vi "line-follower.vi"() -> ()   [LabVIEW 2016]
uses:
  <vilib>/NXT/Block Support/NXT_InputPort.ctl
  <vilib>/NXT/Block Support/NXT_OutputPort.ctl
  <vilib>/NXT/NXTIO Xnodes/NXTIONodeSubVIs/NXTMoveMotors.vi
  <vilib>/NXT/Dual Mode Library/Sensors/EV3_Color_Reflect.vi
  <vilib>/NXT/Dual Mode Library/Waits/Wait_Num(msec).vi
  <vilib>/NXT/NXTIO Xnodes/NXTIONodeSubVIs/NXTStopMotors.vi
  <vilib>/NXT/Dual Mode Library/Waits/Wait_LetGo.vi
  <vilib>/NXT/Dual Mode Library/Waits/Wait_Bump.vi
  <vilib>/NXT/Dual Mode Library/Display/drawText.vi
  <vilib>/NXT/Dual Mode Library/Sensors/Touch_Pressed.vi
  <vilib>/NXT/NXTIO Xnodes/AddressXNode/NXTIOAddress.xnode
  <vilib>/NXT/Subs/LVHSConnector.ctl
  <vilib>/NXT/NXTIO Xnodes/NXTIOXNode/NXTIO.xnode
  <vilib>/NXT/LegoClasses/BrickReference/BrickReference.lvclass
panel:
  out "Counter":sgl
  out "Y":dbl
  out "E":sgl
  out "X":sgl
  out "Motor B":dbl
  out "Motor A":dbl
  out "Avg":sgl
  out "max":sgl
  out "min":sgl
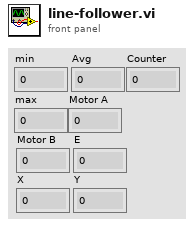
[diagram p1: front panel]
types:
  T1 = typedef "NXT_InputPort.ctl" = u32
  T2 = typedef "NXT_OutputPort.ctl" = u8
  T3 = typedef "LVHSConnector.ctl" = refnum<class "BrickReference.lvclass">
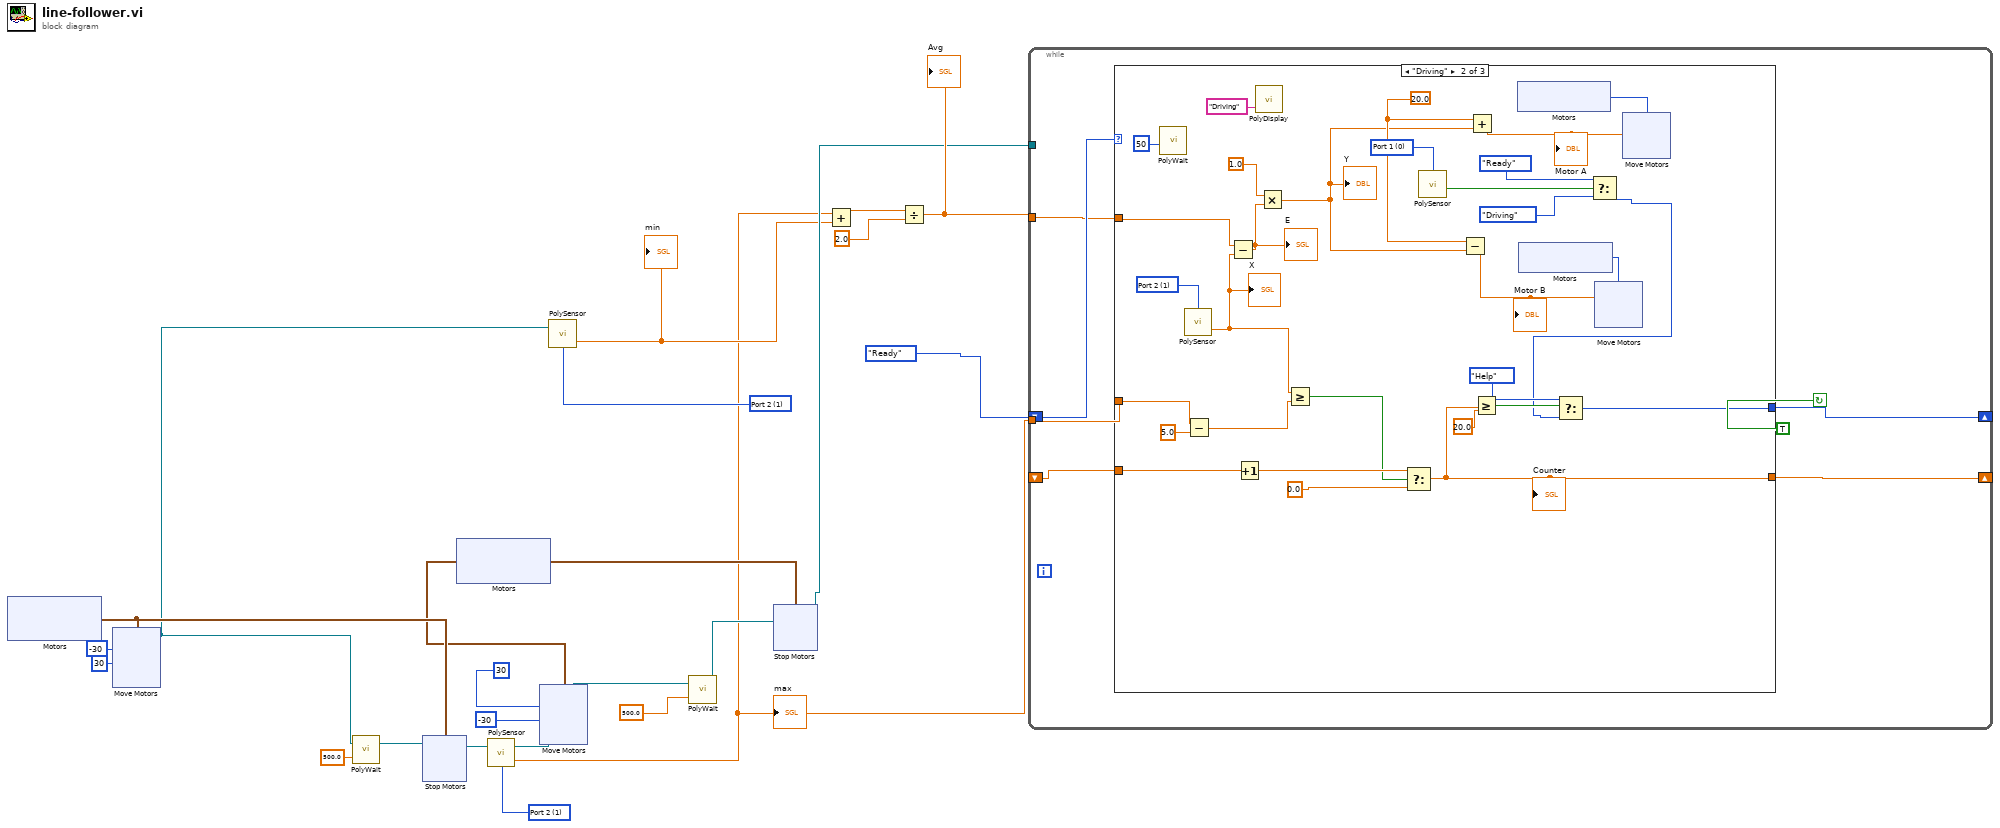
[diagram p0: block diagram]
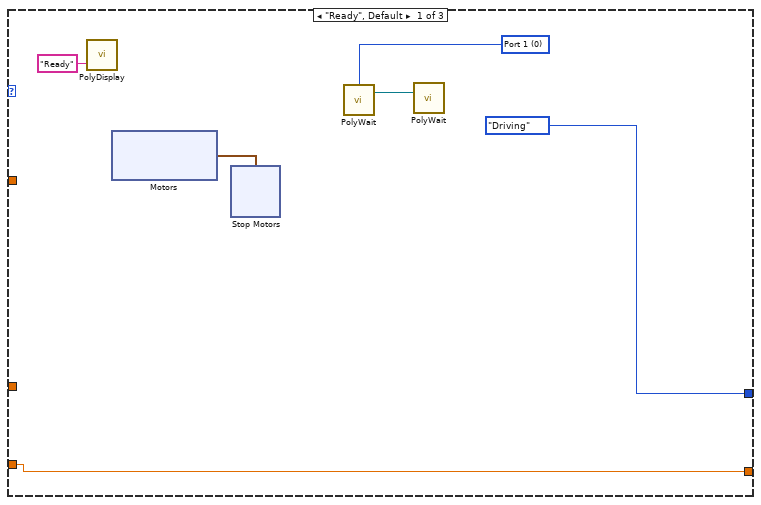
[diagram p2: hidden frame]
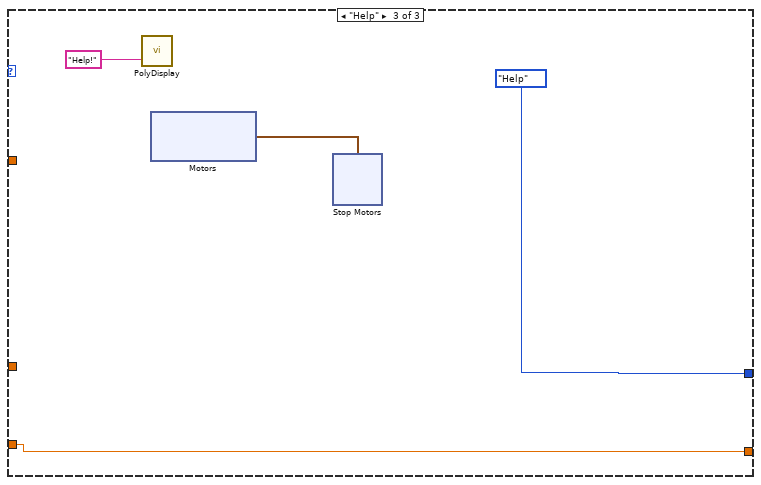
[diagram p3: hidden frame]
diagram:
  w16 = T1 1 items=["Port 1", "Port 2", "Port 3", "Port 4"] ("Port (Port 1)")
  w22 = T1 1 items=["Port 1", "Port 2", "Port 3", "Port 4"] ("Port (Port 1)")
  n1 = xnode "Motors"() -> ("Motor"=w19:cluster{"Port":T2, "Port":T2})
  n2 = xnode "Move Motors"("Power/Speed 2"=i8 30, "Power/Speed 1"=i8 -30, "Motors"=w19) -> ("NXT/EV3"=w14:T3)  [unwired: 1 in]
  n3 = call-poly <vilib>:"PolyWait.vi"("Time (100 msec)"=sgl 500.0 ("Time (1 sec)"), "NXT/EV3"=w14) -> ("NXT/EV3"=w17:T3)  [unwired: 2 in]
  n4 = xnode "Stop Motors"("Motors"=w19, "NXT/EV3"=w17) -> ("NXT/EV3"=w7:T3)
  n5 = xnode "Motors"() -> ("Motor"=w8:cluster{"Port":T2, "Port":T2})
  n6 = call-poly <vilib>:"PolySensor.vi"("NXT/EV3"=w7, "Port (Port 1)"=w16) -> ("Scaled Value"=w1:sgl, "NXT/EV3"=w6:T3)  [unwired: 1 in]
  "max" <- w1
  n7 = xnode "Move Motors"("Power/Speed 2"=i8 -30, "Power/Speed 1"=i8 30, "Motors"=w8, "NXT/EV3"=w6) -> ("NXT/EV3"=w15:T3)
  n8 = call-poly <vilib>:"PolySensor.vi"("NXT/EV3"=w14, "Port (Port 1)"=w22) -> ("Scaled Value"=w4:sgl)  [unwired: 1 in, 1 out]
  "min" <- w4
  n9 = call-poly <vilib>:"PolyWait.vi"("Time (100 msec)"=sgl 500.0 ("Time (1 sec)"), "NXT/EV3"=w15) -> ("NXT/EV3"=w9:T3)  [unwired: 2 in]
  n10 = xnode "Stop Motors"("Motors"=w8, "NXT/EV3"=w9) -> ("NXT/EV3"=w5:T3)
  n11 = Add(x=w1, y=w4) -> (x+y=w3:sgl)
  n12 = Divide(x=w3, y=sgl 2.0) -> (x/y=w10:sgl)
  "Avg" <- w10
  n13 = while {
    tunnel: w10 -> [w28]
    tunnel: w5 -> [_]
    shift-right: [w24] -> _
    shift-left: enum16{"Ready", "Driving", "Help", ""}."Ready" -> [w30]
    tunnel: w1 -> [w27]
    shift-right: [w25] -> _
    shift-left: _ -> [w26]
    stop <- TRUE continue-if-true
    n14 = case shown="\"Driving\"" w30 {
      tunnel: w28 -> [_ w59 _]
      tunnel: w27 -> [_ w58 _]
      tunnel: w26 -> [w32 w54 w92]
      tunnel: [w32 w50 w92] -> w25
      tunnel: [enum16{"Ready", "Driving", "Help", ""}."Driving" w43 enum16{"Ready", "Driving", "Help", ""}."Help"] -> w24
      frame "Ready", Default {
        w36 = T1 0 items=["Port 1", "Port 2", "Port 3", "Port 4"] ("Port (Port 1)")
        n15 = call-poly <vilib>:"PolyDisplay.vi"("Text"="Ready") -> ()  [unwired: 3 in, 1 out]
        n16 = xnode "Motors"() -> ("Motor"=w35:cluster{"Port":T2, "Port":T2})
        n17 = xnode "Stop Motors"("Motors"=w35) -> ()  [unwired: 1 in, 1 out]
        n18 = call-poly <vilib>:"PolyWait.vi"("Port (Port 1)"=w36) -> ("NXTEV3"=w34:T3)  [unwired: 3 in]
        n19 = call-poly <vilib>:"PolyWait.vi"("NXT/EV3"=w34) -> ()  [unwired: 3 in, 1 out]
      }
      frame "Driving" {
        w61 = T1 0 items=["Port 1", "Port 2", "Port 3", "Port 4"] ("Port (Port 1)")
        w64 = T1 1 items=["Port 1", "Port 2", "Port 3", "Port 4"] ("Port (Port 1)")
        w70 = 20.0 ("x")
        n20 = call-poly <vilib>:"PolyWait.vi"("Time (100 msec)"=u32 50) -> ()  [unwired: 3 in, 1 out]
        n21 = call-poly <vilib>:"PolySensor.vi"("Port (Port 1)"=w64) -> ("Scaled Value"=w60:sgl)  [unwired: 2 in, 1 out]
        "X" <- w60
        n22 = Subtract(x=w58, y=sgl 5.0) -> (x-y=w56:sgl)
        n23 = Subtract(x=w59, y=w60) -> (x-y=w72:sgl)
        "E" <- w72
        n24 = Increment(x=w54) -> (x+1=w53:sgl)
        n25 = call-poly <vilib>:"PolyDisplay.vi"("Text"="Driving") -> ()  [unwired: 3 in, 1 out]
        n26 = Multiply(x=1.0, y=w72) -> (x*y=w69:dbl)
        "Y" <- w69
        n27 = Greater Or Equal?(x=w60, y=w56) -> (x >= y?=w51:bool)
        n28 = Select(t=w53, s=w51, f=sgl 0.0 ("y")) -> (s? t:f=w50:sgl)
        "Counter" <- w50
        n29 = call-poly <vilib>:"PolySensor.vi"("Port (Port 1)"=w61) -> ("Yes / No"=w63:bool)  [unwired: 2 in, 1 out]
        n30 = Subtract(x=w70, y=w69) -> (x-y=w67:dbl)
        "Motor B" <- w67
        n31 = Add(x=w70, y=w69) -> (x+y=w68:dbl)
        "Motor A" <- w68
        n32 = Greater Or Equal?(x=w50, y=sgl 20.0) -> (x >= y?=w48:bool)
        n33 = xnode "Motors"() -> ("Motor"=w65:T2)
        n34 = xnode "Motors"() -> ("Motor"=w66:T2)
        n35 = Select(t=enum16{"Ready", "Driving", "Help", ""}."Ready", s=w63, f=enum16{"Ready", "Driving", "Help", ""}."Driving") -> (s? t:f=w44:enum16{"Ready", "Driving", "Help", ""})
        n36 = Select(t=enum16{"Ready", "Driving", "Help", ""}."Help", s=w48, f=w44) -> (s? t:f=w43:enum16{"Ready", "Driving", "Help", ""})
        n37 = xnode "Move Motors"("Power/Speed 1"=w67, "Motors"=w66) -> ()  [unwired: 1 in, 1 out]
        n38 = xnode "Move Motors"("Power/Speed 1"=w68, "Motors"=w65) -> ()  [unwired: 1 in, 1 out]
      }
      frame "Help" {
        n39 = call-poly <vilib>:"PolyDisplay.vi"("Text"="Help!") -> ()  [unwired: 3 in, 1 out]
        n40 = xnode "Motors"() -> ("Motor"=w89:cluster{"Port":T2, "Port":T2})
        n41 = xnode "Stop Motors"("Motors"=w89) -> ()  [unwired: 1 in, 1 out]
      }
    }
  }
